vi "File.Rotate.Manager - Config Dialog.vi"(7 "QName":string="FileRotate", 8 "Error In":errorcluster, 11 "Q In":refnum<queue>) -> (0 "error out":errorcluster, 3 "Qup Q In":refnum<queue>)   [LabVIEW 2024, in "KATE_Lib.lvlib" / "File Utils.lvlib" / "File.Rotate.lvclass"]
uses:
  File.Rotate.lvclass
  Queues/Q.Element.ctl
  Queues/Queue Utils.lvlib
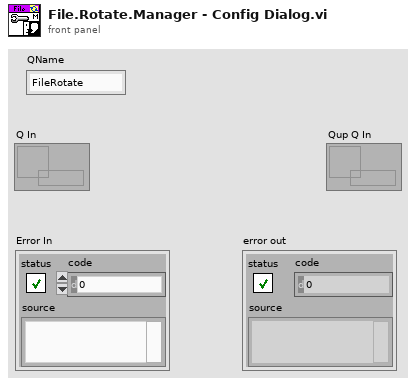
[diagram p1: front panel]
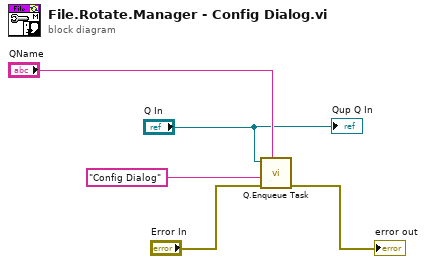
[diagram p0: block diagram]
diagram:
  n1 = call "Q.Enqueue Task.vi"("Q Name"="QName", "Error In"="Error In", "Task Name"="Config Dialog", "Q In"="Q In") -> ("error out"=→"error out":errorcluster)  [unwired: 6 in, 1 out]
  "Qup Q In" <- "Q In"
